vi "PPSU 2 Feedback.vi"(8 "Error in":errorcluster, 11 "All Queue":T1) -> ()   [LabVIEW 2022 SP3]
uses:
  Controls/PPSU 2 Feedback.ctl
  Controls/ALL Health.ctl
  6D_Global.vi
  Controls/All Queue Ref.ctl
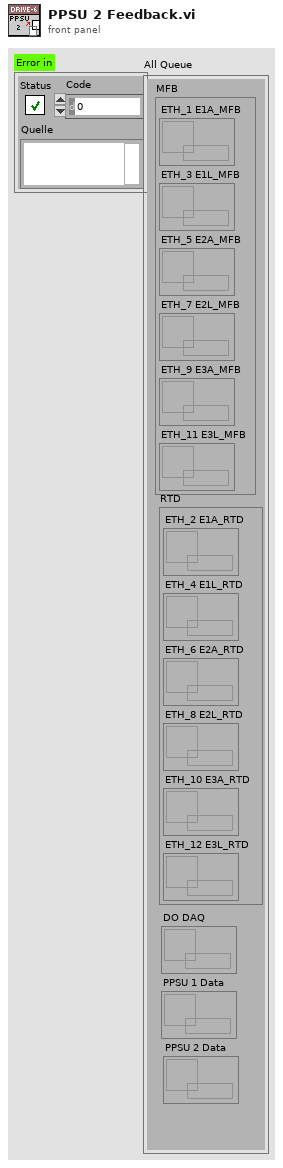
[diagram p1: front panel]
types:
  T1 = typedef "All Queue Ref.ctl" = cluster{"MFB":cluster{"ETH_1 E1A_MFB":refnum<queue>, "ETH_3 E1L_MFB":refnum<queue>, "ETH_5 E2A_MFB":refnum<queue>, "ETH_7 E2L_MFB":refnum<queue>, "ETH_9 E3A_MFB":refnum<queue>, "ETH_11 E3L_MFB":refnum<queue>}, "RTD":cluster{"ETH_2 E1A_RTD ":refnum<queue>, "ETH_4 E1L_RTD ":refnum<queue>, "ETH_6 E2A_RTD ":refnum<queue>, "ETH_8 E2L_RTD ":refnum<queue>, "ETH_10 E3A_RTD ":refnum<queue>, "ETH_12 E3L_RTD ":refnum<queue>}, "DO DAQ":refnum<queue>, "PPSU 1 Data":refnum<queue>, "PPSU 2 Data":refnum<queue>}
  T2 = typedef "PPSU 2 Feedback.ctl" = enum16{"Init", "Poll", "Read", "Exit"}
  T3 = typedef "ALL Health.ctl" = enum16{"DO HS", "Datalog HS", "PPSU HS", "PPSU 2 HS ", "ETH_1", "ETH_2", "ETH_3", "ETH_4", "ETH_5", "ETH_6", "ETH_7", "ETH_8", "ETH_9", "ETH_10", "ETH_11", "ETH_12"}
  T4 = enum16{"Init", "Read 'All'", "Read 'n'", "Read '1'", "Write '1'", "Write 'n'", "Write 'All'"}
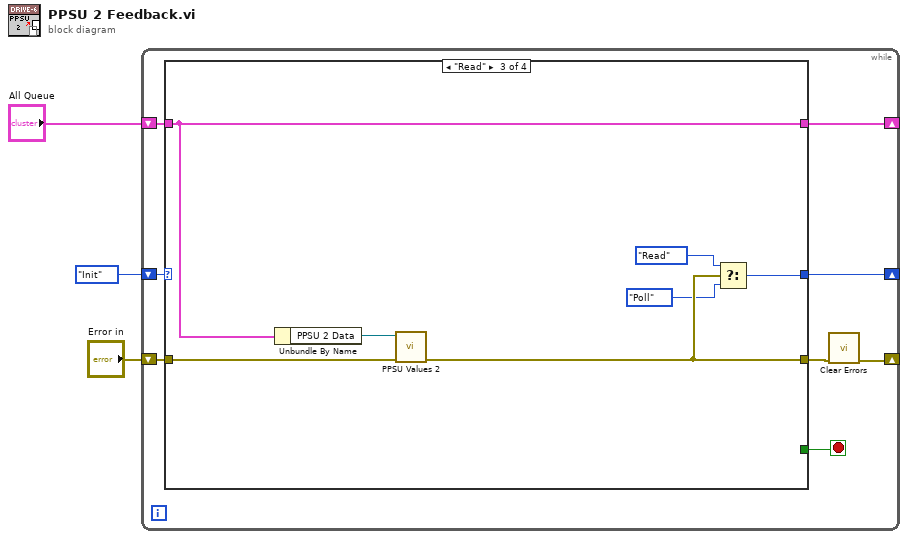
[diagram p0: block diagram]
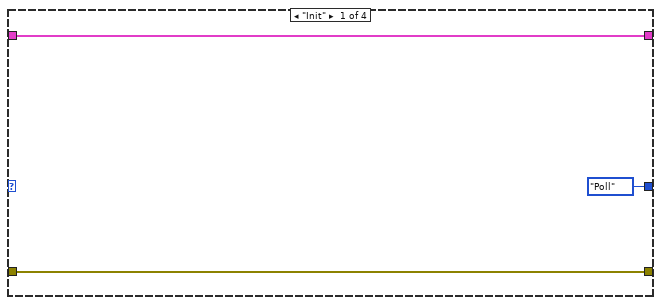
[diagram p2: hidden frame]
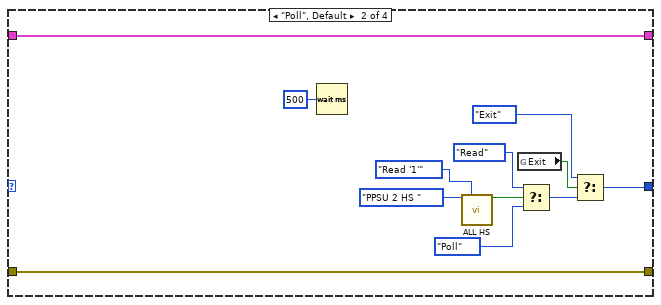
[diagram p3: hidden frame]
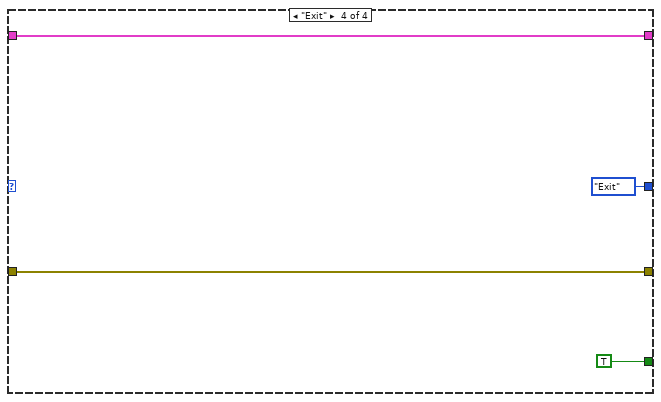
[diagram p4: hidden frame]
diagram:
  n1 = while {
    shift-right: [w10] -> _
    shift-left: PPSU_2_Feedback."Init" -> [w11]
    shift-right: [w7] -> _
    shift-left: "Error in" -> [w9]
    shift-right: [w4] -> _
    shift-left: "All Queue" -> [w5]
    stop <- w6 stop-if-true
    n2 = case shown="\"Read\"" w11 {
      tunnel: [PPSU_2_Feedback."Poll" w21 w32 PPSU_2_Feedback."Exit"] -> w10
      tunnel: w9 -> [w14 w19 w33 w37]
      tunnel: [w14 w19 w31 w37] -> w8
      tunnel: [_ _ _ TRUE] -> w6
      tunnel: w5 -> [w12 w15 w27 w34]
      tunnel: [w12 w15 w27 w34] -> w4
      frame "Init" {
      }
      frame "Poll", Default {
        n3 = Wait (ms)(milliseconds to wait=u32 500) -> ()  [unwired: 1 out]
        n4 = call "ALL HS.vi"("Loop"=ALL_Health."PPSU 2 HS ", "Option"=T4."Read '1'") -> ("Status Out"=w23:bool)  [unwired: 11 in, 2 out]
        n5 = global read "6D_Global.vi" "Exit"() -> (w24:bool)
        n6 = Select(t=PPSU_2_Feedback."Read", s=w23, f=PPSU_2_Feedback."Poll") -> (s? t:f=w22:T2)
        n7 = Select(t=PPSU_2_Feedback."Exit", s=w24, f=w22) -> (s? t:f=w21:T2)
      }
      frame "Read" {
        n8 = Unbundle By Name(w27) -> ("PPSU 2 Data"=w28:refnum<queue>)
        n9 = call "PPSU Values 2.vi"("error in"=w33, "PPSU 2 Q"=w28) -> ("Fehler"=w31:errorcluster)  [unwired: 9 in]
        n10 = Select(t=PPSU_2_Feedback."Read", s=w31, f=PPSU_2_Feedback."Poll") -> (s? t:f=w32:T2)
      }
      frame "Exit" {
      }
    }
    n11 = call <vilib>:"Clear Errors.vi"("error in (no error)"=w8) -> ("error out"=w7:errorcluster)  [unwired: 5 in, 1 out]
  }
